vi "Write State.vi"(8 "error in":errorcluster, 10 "State":bool, 11 "Update Filter State CMD in":refnum<class "Update Filter State CMD.lvclass">) -> (0 "error out":errorcluster, 3 "Update Filter State CMD out":refnum<class "Update Filter State CMD.lvclass">)   [LabVIEW 2014, in "eCRDS Library.lvlib" / "Update Filter State CMD.lvclass"]
uses:
  Update Filter State CMD.lvclass
  Update Filter State CMD.lvclass/Update Filter State CMD.ctl
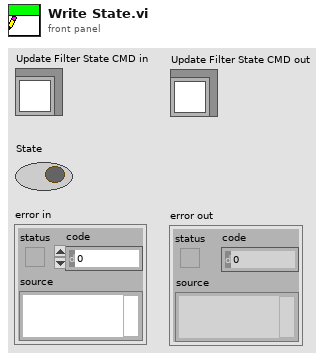
[diagram p1: front panel]
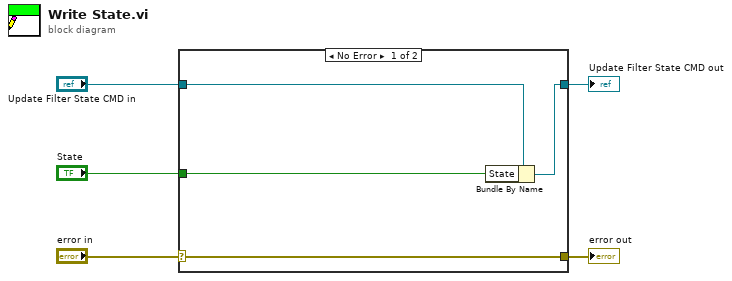
[diagram p0: block diagram]
diagram:
  n1 = case shown="No Error" "error in" {
    selector: "error in" -> [w9 w10]
    tunnel: [w9 w10] -> w4
    tunnel: [w7 w11] -> w2
    tunnel: "Update Filter State CMD in" -> [w8 w11]
    tunnel: "State" -> [w6 _]
    frame No Error {
      n2 = Bundle By Name(cluster=w8, "State"=w6) -> (w7:refnum<class "Update Filter State CMD.lvclass">)
    }
    frame Error {
    }
  }
  "error out" <- w4
  "Update Filter State CMD out" <- w2
